vi "I2C Write.vi"(8 "error in (no error)":errorcluster, 9 "data":u8, 10 "intAddress":u8, 11 "deviceID":u8) -> (0 "error out":errorcluster, 3 "function return":u32)   [LabVIEW 2014, in "atmcd32d.lvlib"]
doc: "unsigned int WINAPI I2CWrite(BYTE deviceID, BYTE intAddress, BYTE data);"
uses:
  atmcd32d.lvlib
  atmcd32d.dll
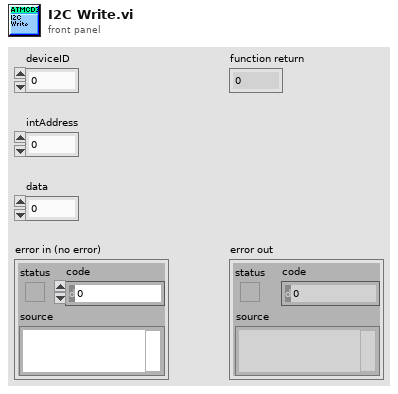
[diagram p1: front panel]
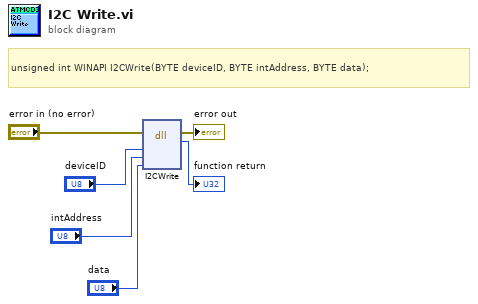
[diagram p0: block diagram]
diagram:
  # "unsigned int WINAPI I2CWrite(BYTE deviceID, BYTE intAddress, BYTE data);"
  n1 = dll-call lib="C:/Users/Bakir/Documents/Lambda2-Testing/lib/Andorlib/atmcd32d.*" fn="I2CWrite"(error in="error in (no error)", "deviceID"="deviceID", "intAddress"="intAddress", "data"="data") -> (error out=→"error out":errorcluster, →"function return":u32)  [unwired: 5 in, 1 out]
